vi "swabian_stream_timetags.vi"(0 "swabian_local_data":T1={"events"={"update_status"=refnum, "update_chart"=refnum, "update_xy"=refnum, "send_channel_data"=refnum}, "stop_q"=refnum, "tagger_reference"=refnum, "connect_button"=refnum, "counter_reference"=refnum, "tagger_stream_reference"=refnum, "log_reference"=refnum, "current_log_offset"=0, "tt20_buffer_q"=refnum, "stream_to_file_button"=refnum, "num_records"=0, "connected?"=FALSE, "plots"=refnum, "histogram_bin_edges"=[], "histogrammer"=refnum, "plot_lifetimes"=refnum, "xy_graph"=refnum, "Reference\nChannel"=enum."ch0", "trigger_channels"=[], "filter_channels"=[], "active_channels"=[], "acq_mode"=0, "Reference\nChannel"=enum."ch0", "acq_time"=0, "sync_period_ps"=0, "raw_stream_path"=path "", "Leftovers"={"missing_sync_data"=[], "missing_events"=0}, "first_batch"=0, "first_sync_stamp"=0, "lifetime_settings"={"Plot Lifetimes"=FALSE, "start_time"=0.0, "stop_time"=0.0, "n_bins"=0, "Oscilloscope"=TRUE}, "Histogram_bins"=[], "last_processed_data"=[], "histogram_data"=[]}, 1 "Data_path":path, 3 "Notes":string="Status: ", 5 "channels_to_stream":bool[](array[boolean])=[FALSE, FALSE, FALSE, FALSE, FALSE, FALSE, FALSE, FALSE], 7 "Trigger edge":bool[](array[boolean])=[FALSE, FALSE, FALSE, FALSE, FALSE, FALSE, FALSE, FALSE], 9 "Reference\nChannel":T3=enum."ch2", 11 "error in (no error)":errorcluster, 12 "acq_time":i64 min=0, 14 "sync_rate":dbl) -> (4 "swabian_local_data 2":T1={"events"={"update_status"=refnum, "update_chart"=refnum, "update_xy"=refnum, "send_channel_data"=refnum}, "stop_q"=refnum, "tagger_reference"=refnum, "connect_button"=refnum, "counter_reference"=refnum, "tagger_stream_reference"=refnum, "log_reference"=refnum, "current_log_offset"=0, "tt20_buffer_q"=refnum, "stream_to_file_button"=refnum, "num_records"=0, "connected?"=FALSE, "plots"=refnum, "histogram_bin_edges"=[], "histogrammer"=refnum, "plot_lifetimes"=refnum, "xy_graph"=refnum, "Reference\nChannel"=enum."ch0", "trigger_channels"=[], "filter_channels"=[], "active_channels"=[], "acq_mode"=0, "Reference\nChannel"=enum."ch0", "acq_time"=0, "sync_period_ps"=0, "raw_stream_path"=path "", "Leftovers"={"missing_sync_data"=[], "missing_events"=0}, "first_batch"=0, "first_sync_stamp"=0, "lifetime_settings"={"Plot Lifetimes"=FALSE, "start_time"=0.0, "stop_time"=0.0, "n_bins"=0, "Oscilloscope"=TRUE}, "Histogram_bins"=[], "last_processed_data"=[], "histogram_data"=[]}, 15 "error out":errorcluster)   [LabVIEW 2018]
uses:
  swabian_local_data_tdef.ctl
  swabian_events_tdef.ctl
  update_chart_tdef.ctl
  channel_data_tdef.ctl
  C:/Users/SWIR TCSPC/Documents/swabian_LV/lib/TTCSharp32.dll
  lib/TTCSharp32.dll
  swabian_buffer_tdef.ctl
  reference_checkbox_tdef.ctl
  lifetime_settings.ctl
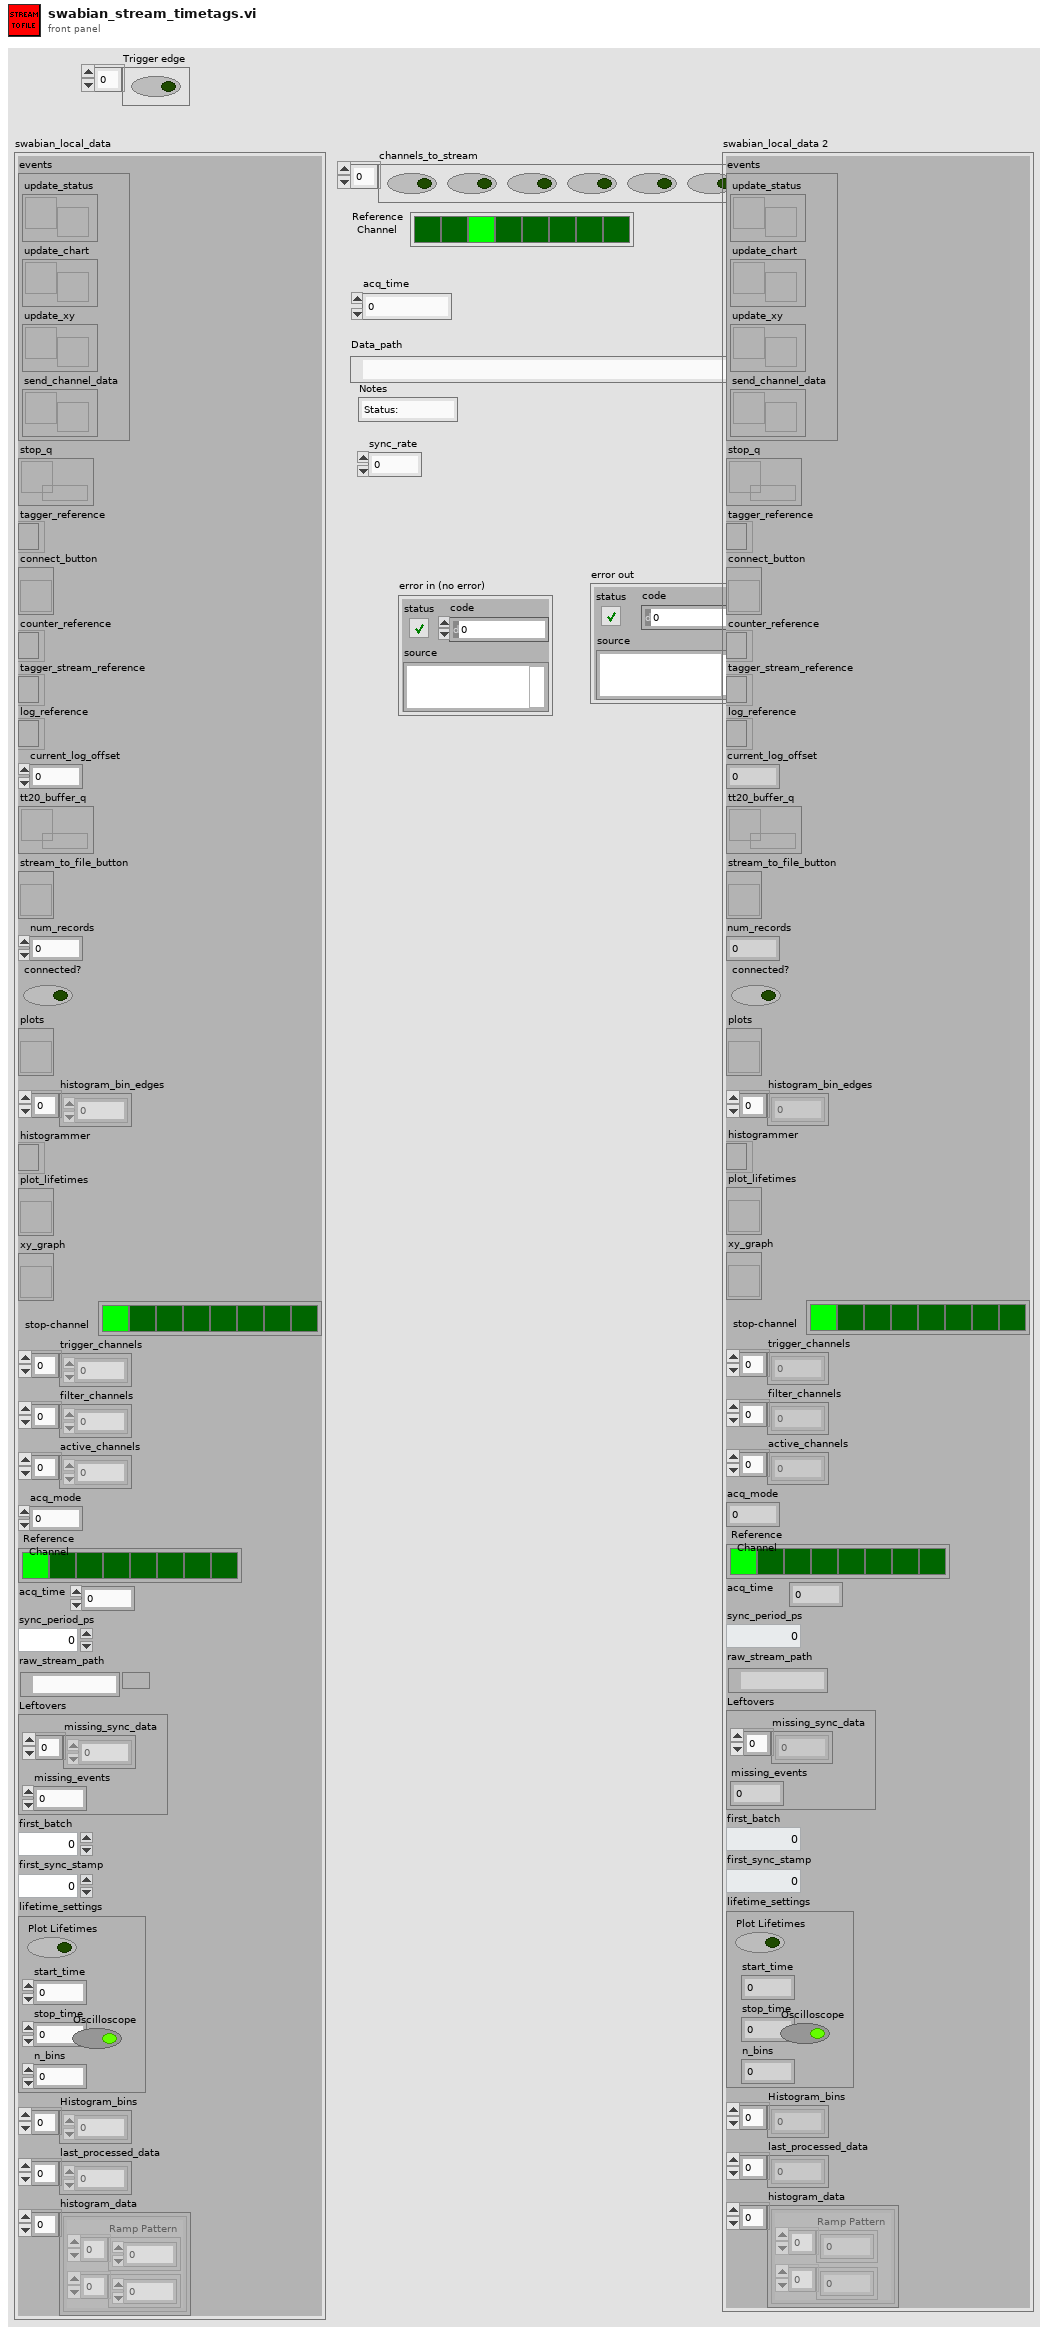
[diagram p1: front panel]
types:
  T1 = typedef "swabian_local_data_tdef.ctl" = cluster{"events":T2, "stop_q":refnum<queue>, "tagger_reference":refnum<k24>, "connect_button":refnum<vi>, "counter_reference":refnum<k24>, "tagger_stream_reference":refnum<k24>, "log_reference":refnum<file>, "current_log_offset":i64, "tt20_buffer_q":refnum<queue>, "stream_to_file_button":refnum<vi>, "num_records":u64, "connected?":bool, "plots":refnum<vi>, "histogram_bin_edges":i64[], "histogrammer":refnum<k24>, "plot_lifetimes":refnum<vi>, "xy_graph":refnum<vi>, "Reference\nChannel":T3, "trigger_channels":i32[], "filter_channels":i32[], "active_channels":i32[], "acq_mode":i32, "Reference\nChannel":T3, "acq_time":i64, "sync_period_ps":i64, "raw_stream_path":path, "Leftovers":cluster{"missing_sync_data":i64[], "missing_events":i32}, "first_batch":i32, "first_sync_stamp":i64, "lifetime_settings":T4, "Histogram_bins":dbl[], "last_processed_data":i64[], "histogram_data":cluster{"Ramp Pattern":dbl[], dbl[]}[]}
  T2 = typedef "swabian_events_tdef.ctl" = cluster{"update_status":refnum<user-event>, "update_chart":refnum<user-event>, "update_xy":refnum<user-event>, "send_channel_data":refnum<user-event>}
  T3 = typedef "reference_checkbox_tdef.ctl" = enum32{"No Selection", "ch0", "ch1", "ch2", "ch3", "ch4", "ch5", "ch6", "ch7"}
  T4 = typedef "lifetime_settings.ctl" = cluster{"Plot Lifetimes":bool, "start_time":dbl, "stop_time":dbl, "n_bins":i32, "Oscilloscope":bool}
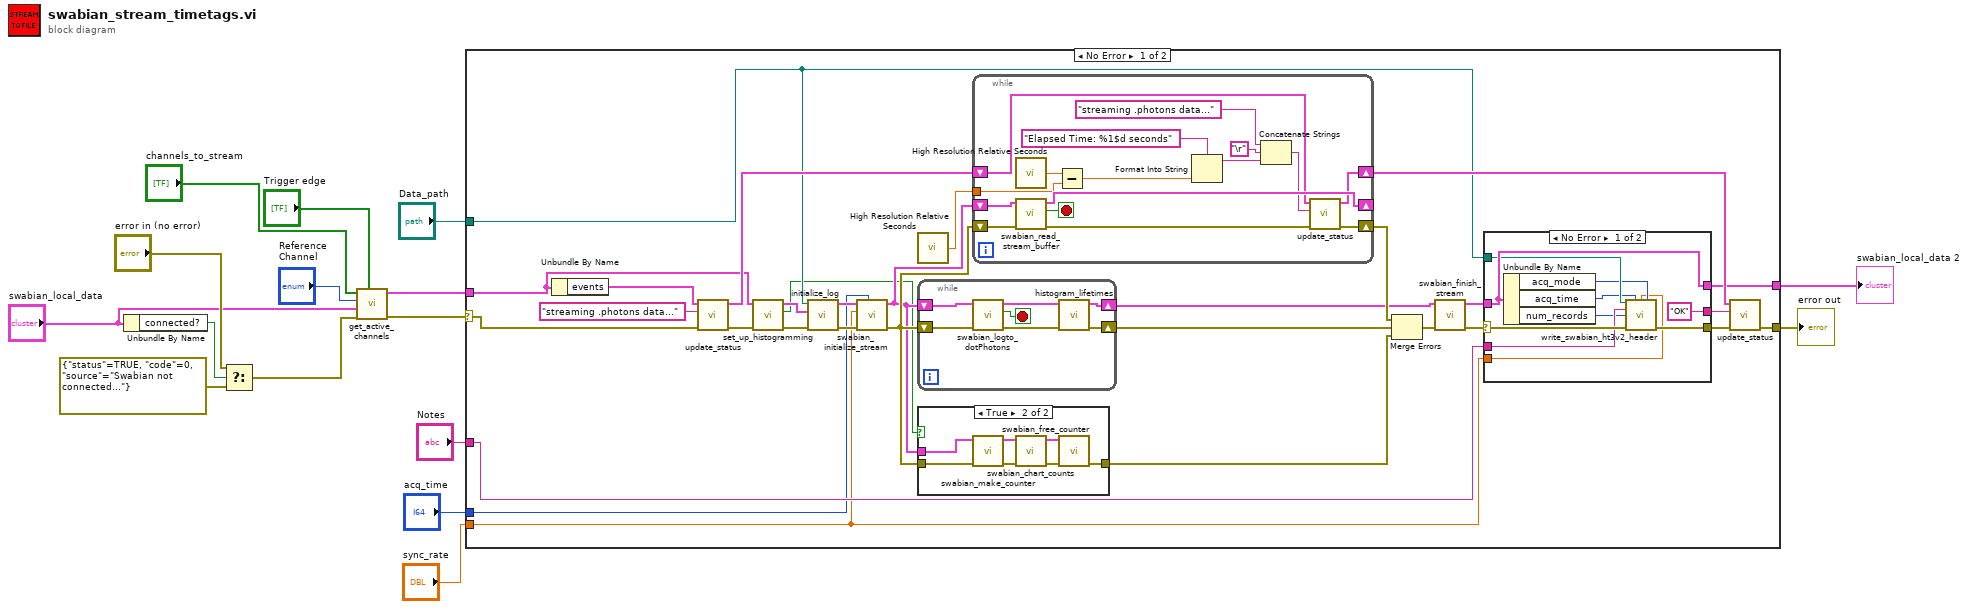
[diagram p0: block diagram]
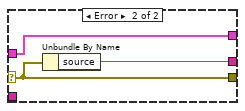
[diagram p3: hidden frame]
diagram:
  n1 = Unbundle By Name("swabian_local_data") -> ("connected?"=w8:bool)
  n2 = Select(t="error in (no error)", s=w8, f=errorcluster {"status"=TRUE, "code"=0, "source"="Swabian not connected..."}) -> (s? t:f=w3:errorcluster)
  n3 = call "get_active_channels.vi"("Trigger edge"="Trigger edge", "Error In"=w3, "swabian_local_data"="swabian_local_data", "Reference\nChannel"="Reference\nChannel", "channels_to_stream"="channels_to_stream") -> ("Error In 2"=w2:errorcluster, "swabian_local_data 2"=w16:T1)  [unwired: 5 in]
  n4 = case shown="No Error" w2 {
    selector: w2 -> [w40 w92]
    tunnel: w16 -> [w19 w91]
    tunnel: "acq_time" -> [w29 _]
    tunnel: "Data_path" -> [w22 _]
    tunnel: [w37 w92] -> w13
    tunnel: [w27 w91] -> w12
    tunnel: "Notes" -> [w30 _]
    tunnel: "sync_rate" -> [w23 _]
    frame No Error {
      n5 = Unbundle By Name(w19) -> ("events"=w39:T2)
      n6 = call "update_status.vi"("error in (no error)"=w40, "status"="streaming .photons data...", "events"=w39) -> ("error out"=w21:errorcluster, "events_out"=w32:T2)  [unwired: 7 in]
      n7 = call "set_up_histogramming.vi"("error in (no error)"=w21, "swabian_local_data 2"=w19) -> ("error out"=w20:errorcluster, "chart_counts?"=w17:bool, "swabian_local_data 3"=w18:T1)  [unwired: 7 in]
      n8 = call "initialize_log.vi"("error in (no error)"=w20, "swabian_local_data 3"=w18, "Data_path"=w22) -> ("error out"=w45:errorcluster, "swabian_local_data 2"=w46:T1)  [unwired: 7 in]
      n9 = call "swabian_initialize_stream.vi"("acq_time"=w29, "error in (no error)"=w45, "sync_rate 2"=w23, "swabian_local_data"=w46) -> ("error out"=w26:errorcluster, "swabian_local_data 2"=w25:T1)  [unwired: 6 in]
      n10 = call <vilib>:"High Resolution Relative Seconds.vi"() -> ("relative seconds"=w33:dbl)
      n11 = while {
        shift-right: [w70] -> w43
        shift-left: w26 -> [w74]
        shift-right: [w68] -> w41
        shift-left: w25 -> [w73]
        stop <- w72 stop-if-true
        n12 = call "swabian_logto_dotPhotons.vi"("error in (no error)"=w74, "swabian_local_data"=w73) -> ("error out"=w71:errorcluster, "stop_loop"=w72:bool, "swabian_local_data 2"=w69:T1)  [unwired: 7 in]
        n13 = call "histogram_lifetimes.vi"("error in (no error)"=w71, "swabian_local_data 2"=w69) -> ("error out"=w70:errorcluster, "swabian_local_data 3"=w68:T1)  [unwired: 8 in]
      }
      n14 = case shown="True" w17 {
        tunnel: w26 -> [w47 w54]
        tunnel: w25 -> [_ w52]
        tunnel: [w47 w48] -> w24
        frame False {
        }
        frame True {
          n15 = call "swabian_make_counter.vi"("error in (no error)"=w54, "swabian_local_data_IN"=w52) -> ("error out"=w53:errorcluster, "swabian_local_data"=w51:T1)  [unwired: 8 in]
          n16 = call "swabian_chart_counts.vi"("error in (no error)"=w53, "swabian_local_data"=w51) -> ("error IO"=w50:errorcluster, "swabian_local_data 2"=w49:T1)  [unwired: 8 in]
          n17 = call "swabian_free_counter.vi"("error in (no error)"=w50, "swabian_local_data_IN"=w49) -> ("error out"=w48:errorcluster)  [unwired: 8 in, 1 out]
        }
      }
      n18 = while {
        shift-right: [w81] -> w44
        shift-left: w26 -> [w89]
        shift-right: [w87] -> _
        shift-left: w25 -> [w88]
        tunnel: w33 -> [w85]
        shift-right: [w75] -> w31
        shift-left: w32 -> [w76]
        stop <- w90 stop-if-true
        n19 = call <vilib>:"High Resolution Relative Seconds.vi"() -> ("relative seconds"=w86:dbl)
        n20 = call "swabian_read_stream_buffer.vi"("error in (no error)"=w89, "swabian_local_data"=w88) -> ("error out"=w82:errorcluster, "stop_loop"=w90:bool, "swabian_local_data 2"=w87:T1)  [unwired: 7 in]
        n21 = Subtract(x=w86, y=w85) -> (x-y=w83:dbl)
        n22 = Format Into String(format string="Elapsed Time: %1$d seconds", w83) -> (resulting string=w78:string)  [unwired: 2 in, 1 out]
        n23 = Concatenate Strings("streaming .photons data..." ("string"), "\r", w78) -> (w77:string)
        n24 = call "update_status.vi"("error in (no error)"=w82, "status"=w77, "events"=w76) -> ("error out"=w81:errorcluster, "events_out"=w75:T2)  [unwired: 7 in]
      }
      n25 = Merge Errors(w44, w43, w24) -> (w42:errorcluster)
      n26 = call "swabian_finish_stream.vi"("error in (no error)"=w42, "swabian_local_data"=w41) -> ("error out"=w36:errorcluster, "swabian_local_data 2"=w28:T1)  [unwired: 8 in]
      n27 = case shown="No Error" w36 {
        selector: w36 -> [w63 w66]
        tunnel: [w62 w66] -> w35
        tunnel: ["OK" ("status") w67] -> w34
        tunnel: w30 -> [w59 _]
        tunnel: w28 -> [w61 w65]
        tunnel: [w61 w65] -> w27
        tunnel: w22 -> [w60 _]
        tunnel: w23 -> [w55 _]
        frame No Error {
          n28 = Unbundle By Name(w61) -> ("acq_mode"=w58:i32, "acq_time"=w57:i64, "num_records"=w56:u64)
          n29 = call "write_swabian_ht3v2_header.vi"("data_path"=w60, "acq_time"=w57, "sync_rate"=w55, "acq_mode"=w58, "data_comment"=w59, "num_records"=w56, "error in (no error)"=w63) -> ("error out"=w62:errorcluster)  [unwired: 8 in]
        }
        frame Error {
          n30 = Unbundle By Name(w66) -> ("source"=w67:string)
        }
      }
      n31 = call "update_status.vi"("error in (no error)"=w35, "status"=w34, "events"=w31) -> ("error out"=w37:errorcluster)  [unwired: 7 in, 1 out]
    }
    frame Error {
    }
  }
  "swabian_local_data 2" <- w12
  "error out" <- w13
